vi "get_installed_app_data.vi"(8 "error in (no error)":errorcluster) -> (0 "error out":errorcluster, 3 "installed_application_data []":T1)   [LabVIEW 2015, in "lv-bin-windows.lvlib" / "v1.lvlib"]
uses:
  v1.lvlib
  <vilib>/registry/registry.llb/Registry RtKey.ctl
  <vilib>/registry/registry.llb/Registry View.ctl
  <vilib>/registry/registry.llb/Registry SAM.ctl
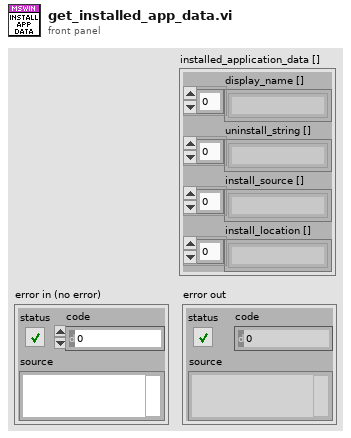
[diagram p1: front panel]
types:
  T1 = cluster{"display_name []":string[], "uninstall_string []":string[], "install_source []":string[], "install_location []":string[]}
  T2 = typedef "Registry SAM.ctl" = enum32{"KEY_QUERY_VALUE", "KEY_SET_VALUE", "KEY_CREATE_SUB_KEY", "KEY_ENUMERATE_SUB_KEYS", "KEY_NOTIFY", "KEY_CREATE_LINK", "KEY_READ", "KEY_WRITE", "KEY_ALL_ACCESS", "KEY_READ | KEY_WRITE"}
  T3 = typedef "Registry View.ctl" = u16
  T4 = typedef "Registry RtKey.ctl" = enum32{"HKEY_CLASSES_ROOT", "HKEY_CURRENT_USER", "HKEY_LOCAL_MACHINE", "HKEY_USERS", "HKEY_PERFORMANCE_DATA", "HKEY_CURRENT_CONFIG", "HKEY_DYN_DATA"}
  T5 = typedef "Registry refnum.ctl" = refnum<k1>
  T6 = cluster{"numSubKeys":i32, "maxSubKeyLen":i32, "maxSubKeyClassLen":i32}
  T7 = cluster{"numValues":i32, "maxValueNameLen":i32, "maxValueDataLen":i32}
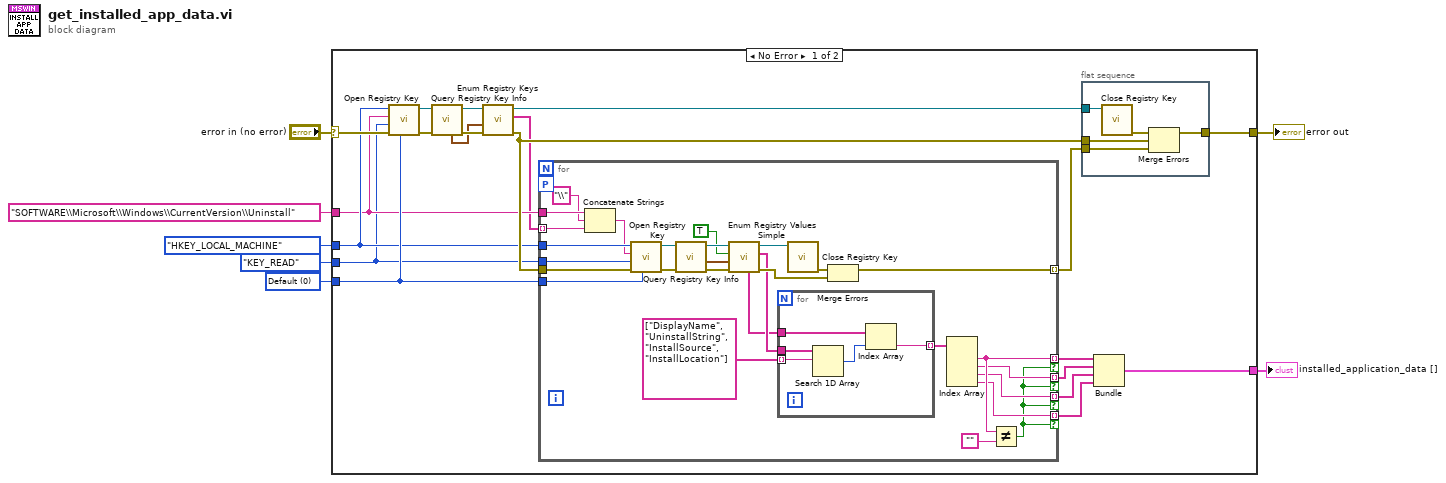
[diagram p0: block diagram]
diagram:
  w7 = T3 0 items=["Default"=0, "KEY_WOW64_64KEY"=8, "KEY_WOW64_32KEY"=9] ("registry view")
  n1 = case shown="No Error" "error in (no error)" {
    selector: "error in (no error)" -> [w26 w66]
    tunnel: w7 -> [w24 _]
    tunnel: Registry_RtKey."HKEY_LOCAL_MACHINE" ("root key (HKEY_LOCAL_MACHINE)") -> [w23 _]
    tunnel: "SOFTWARE\\Microsoft\\Windows\\CurrentVersion\\Uninstall" -> [w17 _]
    tunnel: Registry_SAM."KEY_READ" ("security access mask (KEY_READ | KEY_WRITE)") -> [w14 _]
    tunnel: [w13 w66] -> w2
    tunnel: [w8 _] -> w1
    frame No Error {
      n2 = call <vilib>:"Open Registry Key.vi"("registry view"=w24, "error in (no error)"=w26, "security access mask (KEY_READ | KEY_WRITE)"=w14, "subkey"=w17, "root key (HKEY_LOCAL_MACHINE)"=w23) -> ("error out"=w20:errorcluster, "refnum out"=w22:T5)  [unwired: 5 in]
      n3 = call <vilib>:"Query Registry Key Info.vi"("error in (no error)"=w20, "refnum"=w22) -> ("error out"=w19:errorcluster, "refnum out"=w21:T5, "subkey info"=w18:T6)  [unwired: 5 in, 2 out]
      n4 = call <vilib>:"Enum Registry Keys.vi"("error in (no error)"=w19, "subkey info"=w18, "refnum"=w21) -> ("error out"=w27:errorcluster, "subkeys"=w16:string[], "refnum out"=w25:T5)  [unwired: 6 in]
      n5 = for {
        tunnel: w24 -> [w56]
        tunnel: w23 -> [w55]
        tunnel: w17 -> [w54]
        tunnel: w16 -> [w53] mode=indexing
        tunnel: w14 -> [w41]
        workers-P: _ -> [_]
        tunnel: w27 -> [w57]
        tunnel: [w39] -> w15 mode=indexing
        tunnel: [w37] -> w12 mode=indexing if=w33
        tunnel: [w36] -> w11 mode=indexing if=w33
        tunnel: [w35] -> w10 mode=indexing if=w33
        tunnel: [w34] -> w9 mode=indexing if=w33
        n6 = Concatenate Strings(w54, "\\", w53) -> (w51:string)
        n7 = call <vilib>:"Open Registry Key.vi"("registry view"=w56, "error in (no error)"=w57, "security access mask (KEY_READ | KEY_WRITE)"=w41, "subkey"=w51, "root key (HKEY_LOCAL_MACHINE)"=w55) -> ("error out"=w59:errorcluster, "refnum out"=w58:T5)  [unwired: 5 in]
        n8 = call <vilib>:"Query Registry Key Info.vi"("error in (no error)"=w59, "refnum"=w58) -> ("error out"=w50:errorcluster, "value info"=w47:T7, "refnum out"=w49:T5)  [unwired: 5 in, 2 out]
        n9 = call <vilib>:"Enum Registry Values Simple.vi"("error in (no error)"=w50, "value info"=w47, "retrieve data? (F)"=TRUE, "refnum"=w49) -> ("error out"=w60:errorcluster, "values"=w45:string[], "refnum out"=w48:T5, "String/Binary data"=w44:string[])  [unwired: 2 in, 2 out]
        n10 = for {
          tunnel: w45 -> [w65]
          tunnel: w44 -> [w63]
          tunnel: string[] ["DisplayName", "UninstallString", "InstallSource", "InstallLocation"] -> [w62] mode=indexing
          tunnel: [w61] -> w43 mode=indexing
          n11 = Search 1D Array(1D array=w65, element=w62) -> (index of element=w64:i32)  [unwired: 1 in]
          n12 = Index Array(array=w63, index=w64) -> (element=w61:string)
        }
        n13 = call <vilib>:"Close Registry Key.vi"("refnum"=w48) -> ("error out"=w40:errorcluster)  [unwired: 6 in]
        n14 = Merge Errors(w40, w60) -> (w39:errorcluster)
        n15 = Index Array(array=w43) -> (element #1=w37:string, element #2=w36:string, element #3=w35:string, element #4=w34:string)  [unwired: 4 in]
        n16 = Not Equal?(x=w37, y="") -> (x != y?=w33:bool)
      }
      n17 = flat-sequence {
        tunnel: w25 -> [w32]
        tunnel: w15 -> [w29]
        tunnel: [w30] -> w13
        tunnel: w27 -> [w28]
        frame #0 {
          n18 = call <vilib>:"Close Registry Key.vi"("refnum"=w32) -> ("error out"=w31:errorcluster)  [unwired: 6 in]
          n19 = Merge Errors(w31, w28, w29) -> (w30:errorcluster)
        }
      }
      n20 = Bundle(w12, w11, w10, w9) -> (w8:cluster{string[], string[], string[], string[]})  [unwired: 1 in]
    }
    frame Error {
    }
  }
  "error out" <- w2
  "installed_application_data []" <- w1
